vi "unused_Read size.vi"(8 "error in (no error)":errorcluster, 11 "Terminal In":refnum<class "Terminal.lvclass">) -> (0 "error out":errorcluster, 2 "size":T1, 3 "Terminal Out":refnum<class "Terminal.lvclass">)   [LabVIEW 2023]
uses:
  Terminal.lvclass
  <vilib>/Utility/miscctls.llb/LVBoundsTypeDef.ctl
  Read terminalRef.vi
  Terminal.lvclass/Terminal.ctl
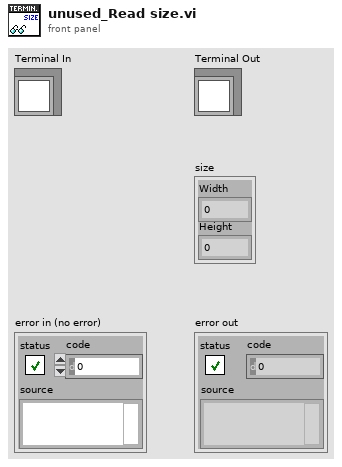
[diagram p1: front panel]
types:
  T1 = typedef "LVBoundsTypeDef.ctl" = cluster{"Width":u32, "Height":u32}
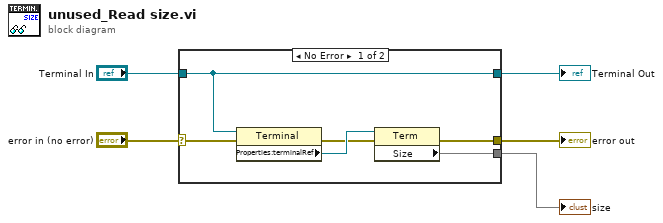
[diagram p0: block diagram]
diagram:
  n1 = case shown="No Error" "error in (no error)" {
    selector: "error in (no error)" -> [w8 w13]
    tunnel: [w7 w13] -> w4
    tunnel: [w11 w12] -> w2
    tunnel: "Terminal In" -> [w11 w12]
    tunnel: [w6 _] -> w1
    frame No Error {
      n2 = property class="Terminal"(reference=w11, error in=w8) -> (error out=w9:errorcluster, "Properties:terminalRef"=w10:refnum<vi>)  [unwired: 1 out]
      n3 = property class="Term"(reference=w10, error in=w9) -> (error out=w7:errorcluster, "Size"=w6)  [unwired: 1 out]
    }
    frame Error {
    }
  }
  "error out" <- w4
  "Terminal Out" <- w2
  "size" <- w1
